vi "write_attributes.vi"(8 "error in (no error)":errorcluster, 10 "attributes":T1, 11 "GaussianMixture in":refnum<class "GaussianMixture.lvclass">) -> (0 "error out":errorcluster, 3 "GaussianMixture out":refnum<class "GaussianMixture.lvclass">)   [LabVIEW 2020, in "GaussianMixture.lvclass"]
uses:
  GaussianMixture.lvclass
  Controls/gaussian_mixture_attributes.ctl
  GaussianMixture.lvclass/GaussianMixture.ctl
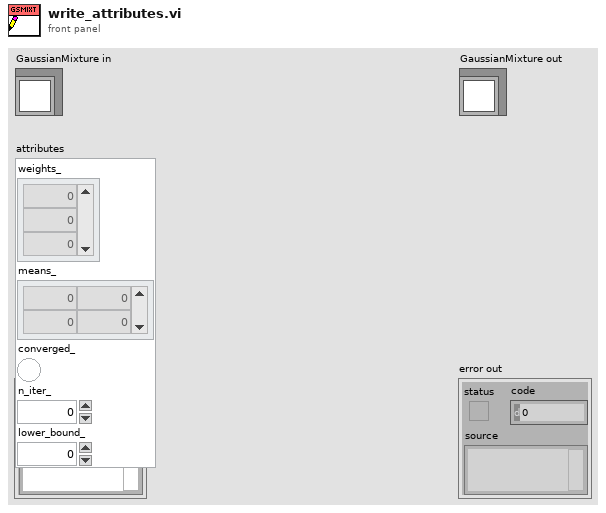
[diagram p1: front panel]
types:
  T1 = typedef "gaussian_mixture_attributes.ctl" = cluster{"weights_":dbl[], "means_":dbl[][], "converged_":bool, "n_iter_":dbl, "lower_bound_":dbl}
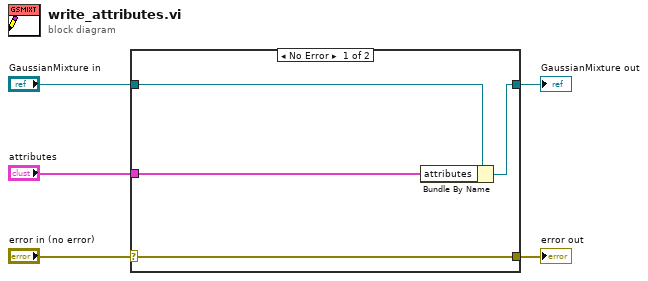
[diagram p0: block diagram]
diagram:
  n1 = case shown="No Error" "error in (no error)" {
    selector: "error in (no error)" -> [w9 w10]
    tunnel: [w9 w10] -> w4
    tunnel: [w7 w11] -> w2
    tunnel: "GaussianMixture in" -> [w8 w11]
    tunnel: "attributes" -> [w6 _]
    frame No Error {
      n2 = Bundle By Name(cluster=w8, "attributes"=w6) -> (w7:refnum<class "GaussianMixture.lvclass">)
    }
    frame Error {
    }
  }
  "error out" <- w4
  "GaussianMixture out" <- w2
